vi "Berechnung mbar.vi"(0 "Volumen in mm³":dbl, 1 "t2":timestamp, 2 "t1":timestamp, 5 "p2":sgl, 7 "p1":sgl, 9 "T2 in C°":sgl, 11 "T1 in C°":sgl, 12 "Fluss in l/min":sgl) -> (4 "n in mbar":sgl format="%#.9f")   [LabVIEW 2020, in "EPA 1065.lvlib" / "Dichtheitstest 1065-345.lvlib"]
uses:
  Dichtheitstest 1065-345.lvlib
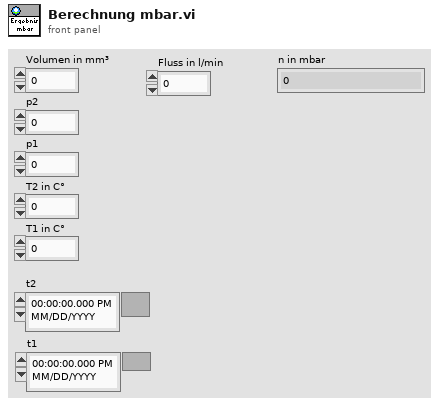
[diagram p1: front panel]
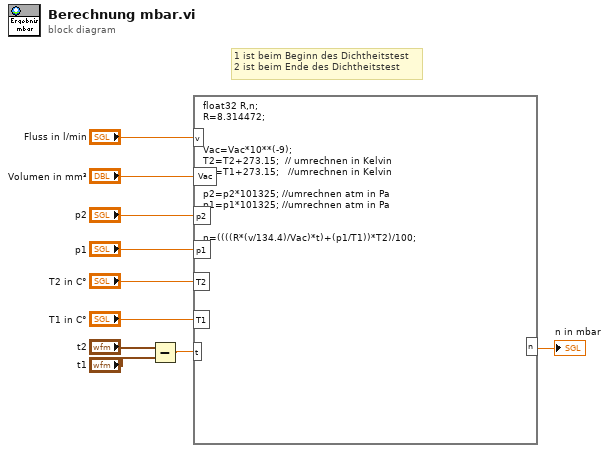
[diagram p0: block diagram]
diagram:
  # "1 ist beim Beginn des Dichtheitstest\n2 ist beim Ende des Dichtheitstest"
  n1 = Subtract(x="t2", y="t1") -> (x-y=w2:dbl)
  n2 = formula code="float32 R,n;\nR=8.314472;\n\n\nVac=Vac*10**(-9);\nT2=T2+273.15;  // umrechnen in Kelvin\nT1=T1+273.15;   //umrechnen in Kelvin\n\np2=p2*101325; //umrechnen atm in Pa\np1=p1*101325; //umrechnen atm in Pa\n\n\nn=((((R*(v/134.4)/Vac)*t)+(p1/T1))*T2)/100;"("Vac"="Volumen in mm³", "p2"="p2", "p1"="p1", "T2"="T2 in C°", "T1"="T1 in C°", "t"=w2, "v"="Fluss in l/min") -> ("n"=→"n in mbar":sgl)
